vi "SeCrTs-AI SEQ MAIN.vi"(8 "error IO":errorcluster) -> (0 "error Out":errorcluster)   [LabVIEW 2022 SP3]
uses:
  RT Controls/ATF Storage-FGV Read write.ctl
  <vilib>/Platform/TimedLoop/XDataNode/wakeup.ctl
  <vilib>/Platform/TimedLoop/XDataNode/XDNodeRunTimeDep.lvlib
  <vilib>/Platform/TimedLoop/XDataNode/nitl_modes.ctl
  <vilib>/Platform/TimedLoop/XDataNode/timing_clust.ctl
  <vilib>/platform/TimedLoop/XDataNode/XDataNode.xnode
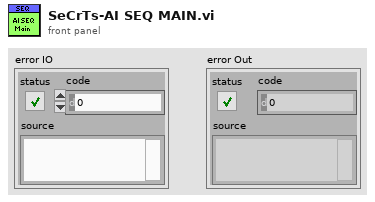
[diagram p1: front panel]
types:
  T1 = typedef "XDNodeRunTimeDep.lvlib/timing_clust.ctl" = cluster{"Expected End [f-1]":u64, "Actual End [f-1]":u64, "Finished Late? [f-1]":bool, "Expected End [i-1]":u64, "Actual End [i-1]":u64, "Finished Late? [i-1]":bool, "Expected Start [i]":u64, "Actual Start [i]":u64, "Expected Start [f]":u64, "Actual Start [f]":u64, "Source Name":string, "Structure Name":string, "Period":i64, "Deadline":i64, "Offset":i64, "Start":i64, "Priority":i32, "Timeout":i32, "Mode":T2, "Wakeup Reason":T3, "Error":errorcluster, "Source Type":string, "Secondary Source Type":string, "Global End Time":u64, "Global Start Time":u64, "Frame Duration":u64, "Iteration Duration":u64, "Assigned CPU":i32, "I/O Scan Engine Mode":u32}
  T2 = typedef "XDNodeRunTimeDep.lvlib/nitl_modes.ctl" = enum32{"No Change", "Process missed periods, maintain original phase", "Discard missed periods, maintain original phase", "Process missed periods, ignore original phase", "Discard missed periods, ignore original phase"}
  T3 = typedef "XDNodeRunTimeDep.lvlib/wakeup.ctl" = enum32{"Normal", "Aborted", "Asynchronous wakeup", "Timing source error", "Timed loop error", "Timeout"}
  T4 = typedef "ATF Storage-FGV Read write.ctl" = enum16{"Write", "Read"}
  T5 = cluster{"Manual HOLD":bool, "Automatic Hold AI":bool, "Abort":bool, "Automatic Hold DI":bool}
  T6 = cluster{"Start DAQ":bool, "Stop DAQ":bool, "RT Stop":bool, "RT Exit":bool, "Start Seq":bool}
  T7 = cluster{cluster{"Sr. No.":string, "Time CDT":string, "Component ID":string, "Data Type":string, "Condition":string, "Range/Position":string, "No of Samples for Pass":string, "Event Duration":string, "Continuous /Cumulative":string, "Expected Delay":string, "Failure case Seq":string, "Current Sequence":string}[]}[]
  T8 = cluster{cluster{"Sr. No.":string, "Time CDT":string, "Component ID":string, "Data Type":string, "Condition":string, "Range/Position":string, "No of Samples for Pass":string, "Event Duration":string, "Continuous /Cumulative":string, "Expected Delay":string, "Failure case Seq":string, "Current Sequence":string}[]}
  T9 = cluster{"Sr. No.":string, "Time CDT":string, "Component ID":string, "Data Type":string, "Condition":string, "Range/Position":string, "No of Samples for Pass":string, "Event Duration":string, "Continuous /Cumulative":string, "Expected Delay":string, "Failure case Seq":string, "Current Sequence":string}[]
  T10 = cluster{"Sr. No.":string, "Time CDT":string, "Component ID":string, "Data Type":string, "Condition":string, "Range/Position":string, "No of Samples for Pass":string, "Event Duration":string, "Continuous /Cumulative":string, "Expected Delay":string, "Failure case Seq":string, "Current Sequence":string}
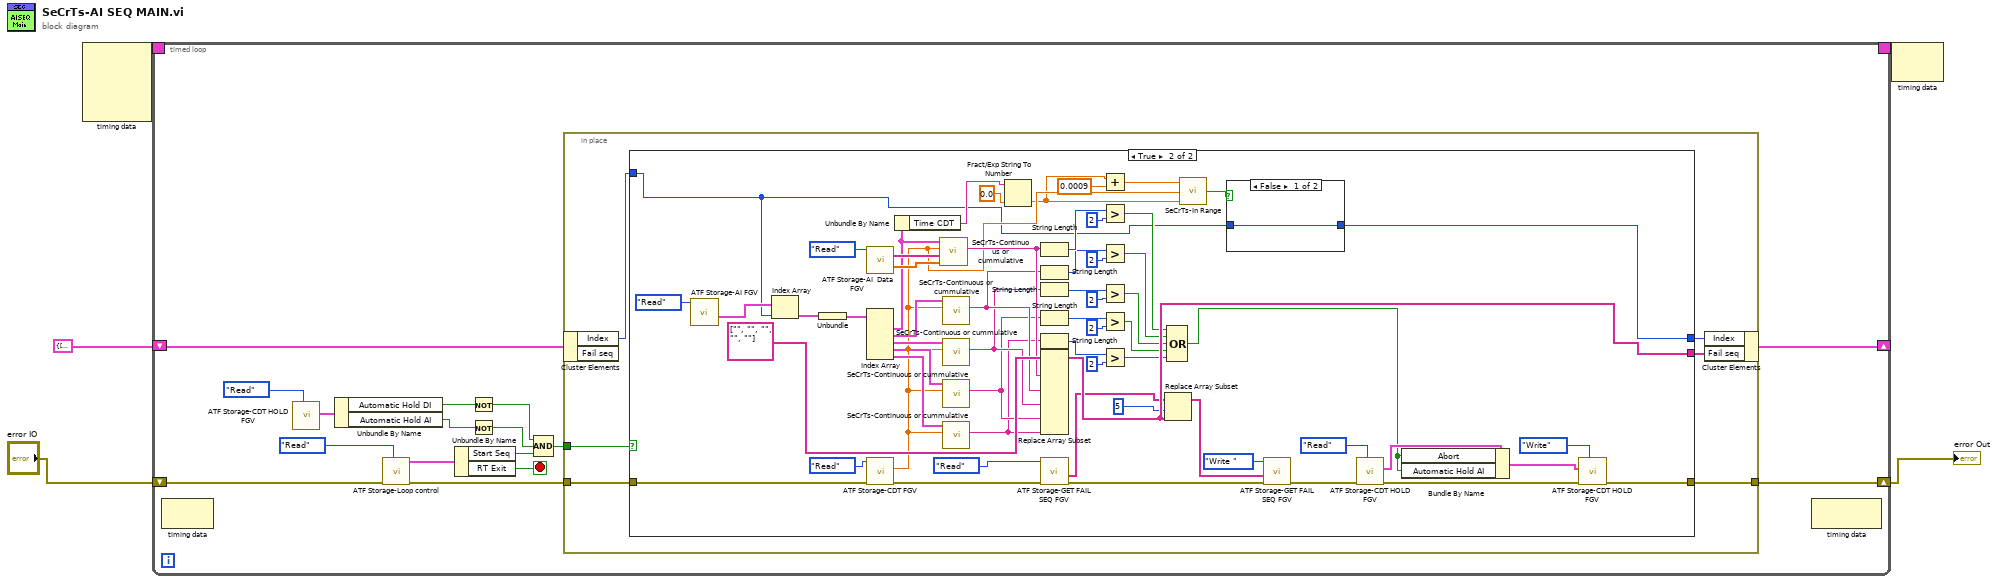
[diagram p0: block diagram]
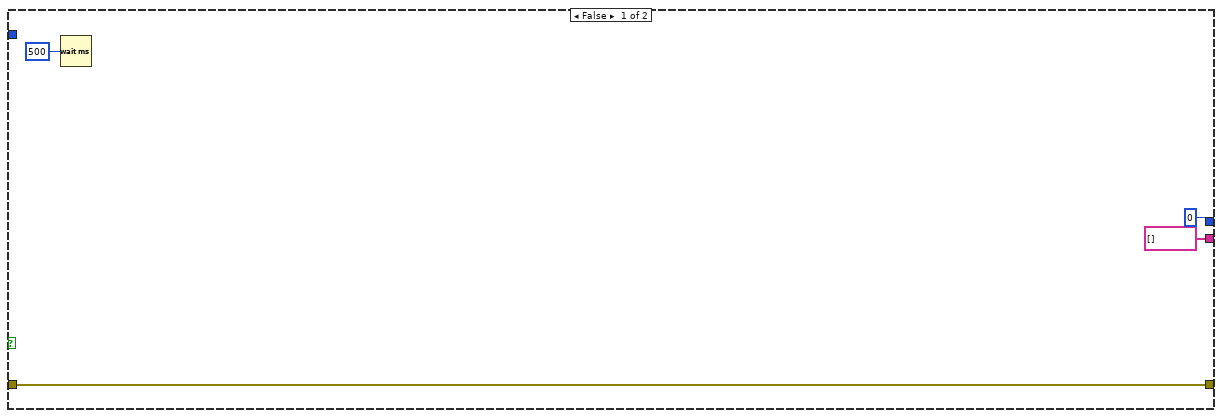
[diagram p2: hidden frame]
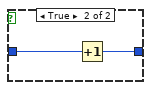
[diagram p3: hidden frame]
diagram:
  n1 = node-c288() -> (w3:T1)  [unwired: 4 in]
  n2 = timed-loop {
    timing: w3 -> [_]
    timing-out: [_] -> w2
    shift-right: [w16] -> w4
    shift-left: "error IO" -> [w12]
    shift-right: [w6] -> _
    shift-left: cluster{"Fail seq":string[], "Index":i32} {"Fail seq"=["", "", "", "", ""], "Index"=0} -> [w7]
    stop <- w8 stop-if-true
    n3 = node-c288() -> ()  [unwired: 1 in, 1 out]
    n4 = call "ATF Storage-CDT HOLD FGV.vi"("Write/Read"=enum16{"Write", "Read"}."Read") -> ("HOLD and Abort Out"=w14:T5)  [unwired: 7 in, 1 out]
    n5 = Unbundle By Name(w14) -> ("Automatic Hold DI"=w18:bool, "Automatic Hold AI"=w19:bool)
    n6 = call "ATF Storage-Loop control.vi"("Action"=enum16{"Init", "Write", "Read"}."Read", "error in (no error)"=w12) -> ("error Out"=w11:errorcluster, "Loop Control out"=w10:T6)  [unwired: 8 in]
    n7 = Unbundle By Name(w10) -> ("Start Seq"=w9:bool, "RT Exit"=w8:bool)
    n8 = Not(x=w18) -> (.not. x?=w17:bool)
    n9 = Not(x=w19) -> (.not. x?=w21:bool)
    n10 = Compound Arithmetic op=AND(w17, w21, w9) -> (w20:bool)
    n11 = in-place {
      in-place-border: [w27] -> w16
      in-place-border: w20 -> [w26]
      in-place-border: w11 -> [w25]
      n12 = in-place-cluster #1(w7) -> ("Index"=w24:i32)  [unwired: 1 out]
      n13 = case shown="True" w26 {
        tunnel: w25 -> [w31 w91]
        tunnel: [w31 w88] -> w27
        tunnel: w24 -> [_ w32]
        tunnel: [0 ("Index") w87] -> w23
        tunnel: [string[] [] ("array") w86] -> w22
        frame False {
          n14 = Wait (ms)(milliseconds to wait=u32 500) -> ()  [unwired: 1 out]
        }
        frame True {
          n15 = call "ATF Storage-AI FGV.vi"("Enum"=enum16{"Read", "Write "}."Read") -> ("AI Seq  Out"=w34:T7)  [unwired: 9 in, 1 out]
          n16 = Index Array(array=w34, index=w32) -> (element=w33:T8)
          n17 = Unbundle(w33) -> (w81:T9)
          n18 = call "ATF Storage-AI  Data  FGV.vi"("Write/Read"=ATF_Storage-FGV_Read_write."Read") -> ("AI Channels Name LP"=w79:string[], "AI Y LP data"=w78:dbl[])  [unwired: 11 in, 2 out]
          n19 = Index Array(array=w81) -> (element #1=w42:T10, element #2=w84:T10, element #3=w83:T10, element #4=w82:T10, element #5=w75:T10)  [unwired: 5 in]
          n20 = call "ATF Storage-CDT FGV.vi"("error in (no error)"=w91, "Write/Read"=enum16{"Write", "Read"}."Read") -> ("error Out"=w74:errorcluster, "CDT Out"=w38:dbl)  [unwired: 8 in]
          n21 = Unbundle By Name(w42) -> ("Time CDT"=w40:string)
          n22 = call "SeCrTs-Continuous or cummulative.vi"("AI  data"=w78, "AI Channels Name LP"=w79, "CDT"=w38, "output cluster"=w42) -> ("Failure case Seq"=w72:string)  [unwired: 6 in, 1 out]
          n23 = call "SeCrTs-Continuous or cummulative.vi"("CDT"=w38, "output cluster"=w84) -> ("Failure case Seq"=w67:string)  [unwired: 8 in, 1 out]
          n24 = call "SeCrTs-Continuous or cummulative.vi"("CDT"=w38, "output cluster"=w83) -> ("Failure case Seq"=w60:string)  [unwired: 8 in, 1 out]
          n25 = call "SeCrTs-Continuous or cummulative.vi"("CDT"=w38, "output cluster"=w82) -> ("Failure case Seq"=w59:string)  [unwired: 8 in, 1 out]
          n26 = call "SeCrTs-Continuous or cummulative.vi"("CDT"=w38, "output cluster"=w75) -> ("Failure case Seq"=w57:string)  [unwired: 8 in, 1 out]
          n27 = Fract/Exp String To Number(string=w40, default (0 dbl)=0.0) -> (number=w36:dbl)  [unwired: 2 in, 1 out]
          n28 = String Length(string=w72) -> (length=w71:i32)
          n29 = String Length(string=w67) -> (length=w68:i32)
          n30 = String Length(string=w60) -> (length=w61:i32)
          n31 = String Length(string=w59) -> (length=w63:i32)
          n32 = String Length(string=w57) -> (length=w58:i32)
          n33 = Replace Array Subset(array=string[] ["", "", "", "", ""], new element #1=w72, new element #2=w67, new element #3=w60, new element #4=w59, new element #5=w57) -> (w86:string[])  [unwired: 5 in]
          n34 = call "ATF Storage-GET FAIL SEQ FGV.vi"("error in"=w74, "Enum"=enum16{"Read", "Write "}."Read") -> ("error out"=w73:errorcluster, "Failure \ncase Seq"=w66:string[])  [unwired: 8 in]
          n35 = Add(x=w36, y=0.0009) -> (x+y=w37:dbl)
          n36 = Greater?(x=w71, y=2) -> (0:w55:bool)
          n37 = Greater?(x=w68, y=2) -> (0:w54:bool)
          n38 = Greater?(x=w61, y=2) -> (0:w53:bool)
          n39 = Greater?(x=w63, y=2) -> (0:w52:bool)
          n40 = Greater?(x=w58, y=2) -> (0:w51:bool)
          n41 = Replace Array Subset(array=w66, new element=w86, index=5) -> (w64:string[])
          n42 = Compound Arithmetic op=OR(w55, w54, w53, w52, w51) -> (w43:bool)
          n43 = call "SeCrTs-In Range.vi"("Min"=w36, "X"=w38, "Max"=w37) -> ("In Range"=w39:bool)  [unwired: 2 in]
          n44 = case shown="False" w39 {
            tunnel: w32 -> [w92 w94]
            tunnel: [w92 w93] -> w87
            frame False {
            }
            frame True {
              n45 = Increment(x=w94) -> (x+1=w93:i32)
            }
          }
          n46 = call "ATF Storage-GET FAIL SEQ FGV.vi"("error in"=w73, "Failure \ncase Seq"=w64, "Enum"=enum16{"Read", "Write "}."Write ") -> ("error out"=w47:errorcluster)  [unwired: 7 in, 1 out]
          n47 = call "ATF Storage-CDT HOLD FGV.vi"("Write/Read"=enum16{"Write", "Read"}."Read", "error in (no error)"=w47) -> ("error Out"=w46:errorcluster, "HOLD and Abort Out"=w45:T5)  [unwired: 6 in]
          n48 = Bundle By Name(cluster=w45, "Abort"=w43, "Automatic Hold AI"=w43) -> (w44:T5)
          n49 = call "ATF Storage-CDT HOLD FGV.vi"("Write/Read"=enum16{"Write", "Read"}."Write", "error in (no error)"=w46, "HOLD and Abort"=w44) -> ("error Out"=w88:errorcluster)  [unwired: 5 in, 1 out]
        }
      }
      n50 = in-place-cluster #1("Index"=w23, "Fail seq"=w22) -> (w6:cluster{"Fail seq":string[], "Index":i32})
    }
    n51 = node-c288() -> ()  [unwired: 1 in, 1 out]
  }
  "error Out" <- w4
  n52 = node-c288(w2) -> ()  [unwired: 1 out]
